vi "subscribe event.vi"(6 "publishing module ID":string, 7 "subscribing module ID":string, 8 "error in":errorcluster, 9 "published element":string, 10 "subscribed element":string, 11 "engine configuration in":refnum<class "engine configuration.lvclass">) -> (0 "error out":errorcluster, 3 "engine configuration out":refnum<class "engine configuration.lvclass">)   [LabVIEW 2013, in "engine configuration.lvclass"]
uses:
  engine configuration.lvclass
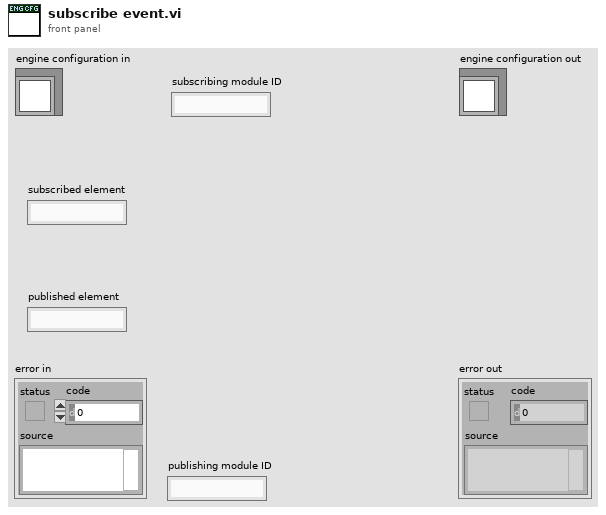
[diagram p1: front panel]
types:
  T1 = typedef "engine configuration.lvclass/simple mapping.ctl" = cluster{"module ID":string[], "publisher":string[], "subscribers":T2[]}
  T2 = typedef "engine configuration.lvclass/module channel pairings.ctl" = cluster{"modules":string[], "element":string[]}
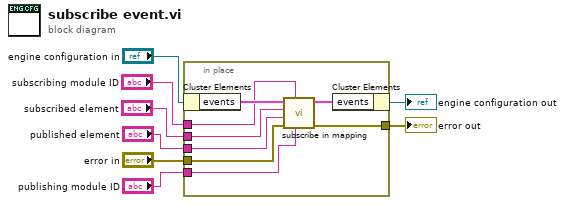
[diagram p0: block diagram]
diagram:
  n1 = in-place {
    in-place-border: "error in" -> [w13]
    in-place-border: "subscribing module ID" -> [w11]
    in-place-border: "subscribed element" -> [w15]
    in-place-border: [w14] -> w3
    in-place-border: "publishing module ID" -> [w10]
    in-place-border: "published element" -> [w9]
    n2 = in-place-cluster #1("engine configuration in") -> ("events"=w12:T1)
    n3 = call "subscribe in mapping.vi"("publishing module ID"=w10, "subscribing module ID"=w11, "error in"=w13, "published element"=w9, "subscribed element"=w15, "mappings in"=w12) -> ("error out"=w14:errorcluster, "mappings out"=w16:T1)  [unwired: 4 in]
    n4 = in-place-cluster #1("events"=w16) -> (→"engine configuration out":refnum<class "engine configuration.lvclass">)
  }
  "error out" <- w3
